vi "2DArray2WaveForm_FileWarite.vi"() -> ()   [LabVIEW 2023]
panel:
  out "Waveform Graph":waveform(dbl)[](graph)
  out "Waveform Chart":waveform(dbl)[](graph)
  in  "Array 3":dbl[][](array[numeric])
  out "Array 2":waveform(dbl)[](array[waveform])
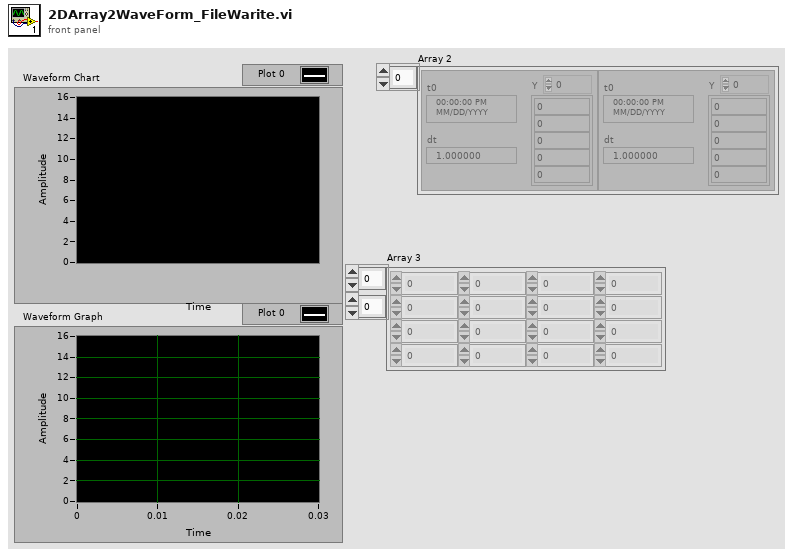
[diagram p1: front panel]
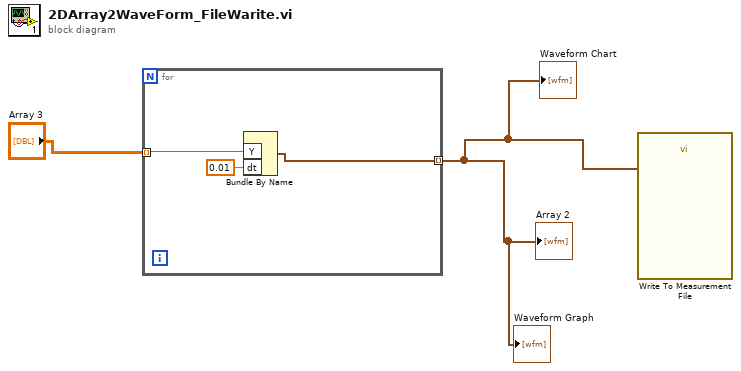
[diagram p0: block diagram]
diagram:
  n1 = for {
    tunnel: [w4] -> w1 mode=indexing
    tunnel: "Array 3" -> [w3] mode=indexing
    n2 = Bundle By Name("Y"=w3, "dt"=0.01) -> (w4:waveform(dbl))  [unwired: 1 in]
  }
  "Array 2" <- w1
  "Waveform Chart" <- w1
  "Waveform Graph" <- w1
  n3 = call "Write To Measurement File"("Signals"=w1) -> ()  [unwired: 16 in, 3 out]
